vi "setConnected.vi"(8 "error in (no error)":errorcluster, 10 "connected":bool, 11 "TCPConnection in":refnum<class "TCPConnection.lvclass">) -> (0 "error out":errorcluster, 3 "TCPConnection out":refnum<class "TCPConnection.lvclass">)   [LabVIEW 2013]
uses:
  TCPConnection.lvclass
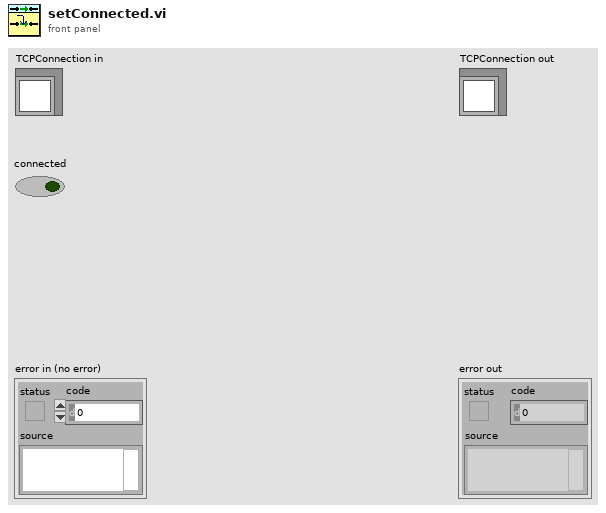
[diagram p1: front panel]
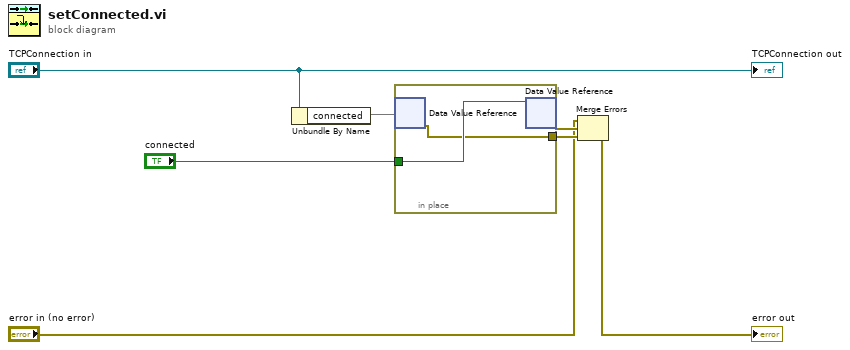
[diagram p0: block diagram]
diagram:
  n1 = Unbundle By Name("TCPConnection in") -> ("connected"=w6)
  n2 = in-place {
    in-place-border: "connected" -> [w9]
    in-place-border: [w8] -> w3
    n3 = in-place-dvr #1(w6) -> (w8:errorcluster)  [unwired: 1 out]
    n4 = in-place-dvr #1(w9) -> (w4:errorcluster)  [unwired: 1 out]
  }
  n5 = Merge Errors("error in (no error)", w4, w3) -> (→"error out":errorcluster)
  "TCPConnection out" <- "TCPConnection in"
